vi "Event Handler.vi"(8 "error in (no error)":errorcluster, 10 "Stop Event Handler":refnum<user-event>, 11 "TreeDirectory in":refnum<class "TreeDirectory.lvclass">) -> (0 "error out":errorcluster)   [LabVIEW 2015, in "TreeDirectory.lvclass"]
doc: "The <b>Event Handler VI</b> is a dynamic dispatch VI that should be overwritten if events are needed to create the enhanced QControl. \n\nBy inheriting from the main Control.lvclass the overwritten <b>Event Handler VI</b> will be launched asynchronously in the initialization of the QControl.\n<b> </b> <b> </b>\n©2016 Q Software Innovations, LLC (QSI)\nwritten by Quentin Alldredge\nproduced in LabVIEW 2015\n\nsupport@qsoftwareinnovations.com\nwww.qsoftwareinnovations.com\n\nAll rights reserved.\n\nRedistribution and use in source and binary forms, with or without modification, are permitted provided that the following conditions are met:\n\n * Redistributions of source code must retain the above copyright notice, this list of conditions and the following disclaimer.\n * Redistributions in binary form must reproduce the above copyright notice, this list of conditions and the following disclaimer in the documentation and/or other materials provided with the distribution.\n * Neither the name of Q Software Innovations, LLC. nor the names of its contributors may be used to endorse or promote products derived from this software without specific prior written permission.\n\nTHIS SOFTWARE IS PROVIDED BY THE COPYRIGHT HOLDERS AND CONTRIBUTORS \"AS IS\" AND ANY EXPRESS OR IMPLIED WARRANTIES, INCLUDING, BUT NOT LIMITED TO, THE IMPLIED WARRANTIES OF MERCHANTABILITY AND FITNESS FOR A PARTICULAR PURPOSE ARE DISCLAIMED. IN NO EVENT SHALL THE COPYRIGHT OWNER OR CONTRIBUTORS BE LIABLE FOR ANY DIRECT, INDIRECT, INCIDENTAL, SPECIAL, EXEMPLARY, OR CONSEQUENTIAL DAMAGES (INCLUDING, BUT NOT LIMITED TO, PROCUREMENT OF SUBSTITUTE GOODS OR SERVICES; LOSS OF USE, DATA, OR PROFITS; OR BUSINESS INTERRUPTION) HOWEVER CAUSED AND ON ANY THEORY OF LIABILITY, WHETHER IN CONTRACT, STRICT LIABILITY, OR TORT (INCLUDING NEGLIGENCE OR OTHERWISE) ARISING IN ANY WAY OUT OF THE USE OF THIS SOFTWARE, EVEN IF ADVISED OF THE POSSIBILITY OF SUCH DAMAGE."
uses:
  TreeDirectory.lvclass
  TreeDirectory.lvclass/TreeDirectory.ctl
  TreeControl/TreeControl.lvclass
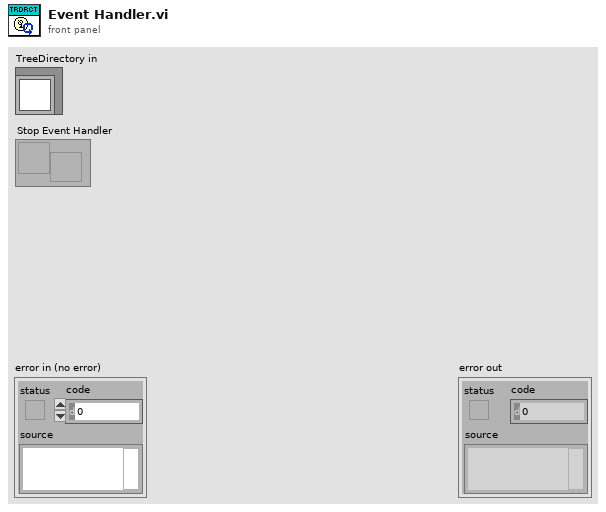
[diagram p1: front panel]
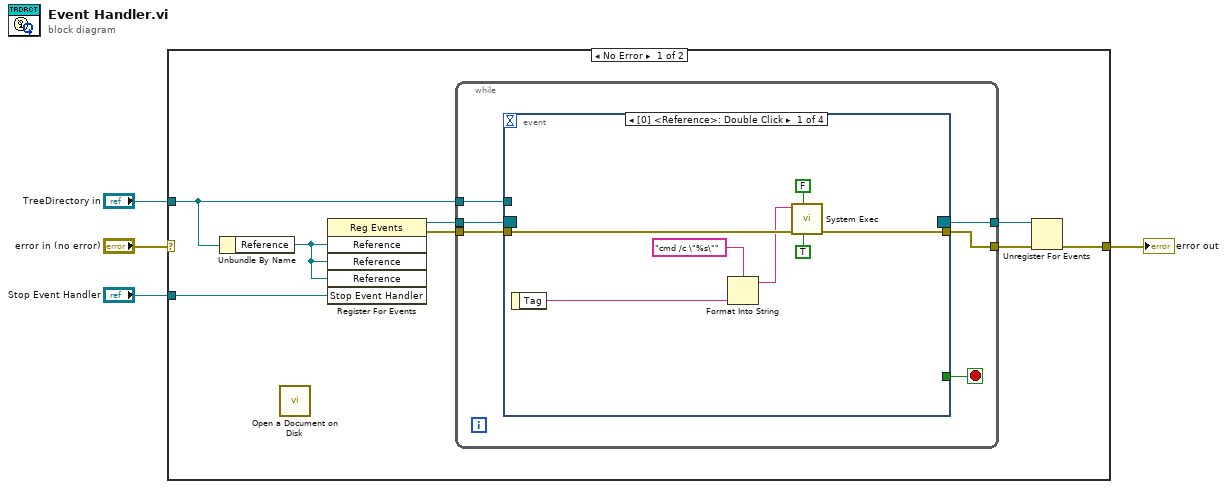
[diagram p0: block diagram]
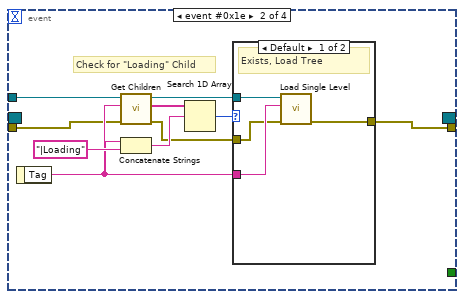
[diagram p2: hidden frame]
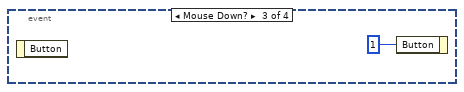
[diagram p4: hidden frame]
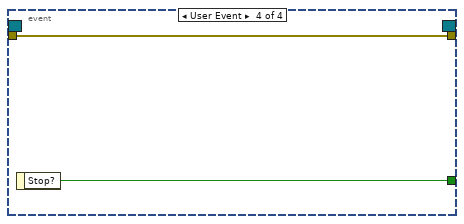
[diagram p5: hidden frame]
diagram:
  n1 = case shown="No Error" "error in (no error)" {
    selector: "error in (no error)" -> [_ w44]
    tunnel: [w9 w44] -> w3
    tunnel: "TreeDirectory in" -> [w7 _]
    tunnel: "Stop Event Handler" -> [w6 _]
    frame No Error {
      n2 = Unbundle By Name(w7) -> ("Reference"=w5:refnum<vi>)
      n3 = call <vilib>:"Open a Document on Disk.vi"() -> ()  [unwired: 7 in, 1 out]
      n4 = register-events(w5, w5, w5, w6) -> (reference out=w12:refnum<event-registration>, error out=w11:errorcluster)  [unwired: 2 in]
      n5 = while {
        tunnel: w12 -> [w18]
        tunnel: w11 -> [w16]
        tunnel: [w15] -> w10
        tunnel: [w13] -> w8
        tunnel: w7 -> [w17]
        stop <- w14 stop-if-true
        n6 = event shown="[0] <Reference>: Double Click" {
          selector: w18 -> [_ _ _ _]
          dyn-events: [_ _ _ _] -> w13
          timeout: _ -> [_ _ _ _]
          tunnel: w17 -> [_ w35 _ _]
          tunnel: w16 -> [w25 w28 _ w43]
          tunnel: [w24 w26 _ w43] -> w15
          tunnel: [_ _ _ w42] -> w14
          event Double Click {
            n7 = event-data() -> ("Tag"=w23:string)  [unwired: 1 in]
            n8 = Format Into String(format string="cmd /c \"%s\"", w23) -> (resulting string=w21:string)  [unwired: 2 in, 1 out]
            n9 = call <vilib>:"System Exec.vi"("run minimized? (F)"=TRUE, "wait until completion? (T)"=FALSE, "error in (no error)"=w25, "command line"=w21) -> ("error out"=w24:errorcluster)  [unwired: 4 in, 3 out]
          }
          event event #0x1e {
            # "Check for \"Loading\" Child"
            n10 = event-data() -> ("Tag"=w29:string)  [unwired: 1 in]
            n11 = call "Get Children.vi"("error in (no error)"=w28, "Tag"=w29, "Tree in"=w35) -> ("error out"=w27:errorcluster, "ChildrenTags[]"=w33:string[], "Tree out"=w30:refnum<class "TreeDirectory.lvclass">)  [unwired: 6 in]
            n12 = Concatenate Strings(w29, "|Loading" ("string")) -> (w32:string)
            n13 = Search 1D Array(1D array=w33, element=w32) -> (index of element=w31:i32)  [unwired: 1 in]
            n14 = case shown="Default" w31 {
              tunnel: w30 -> [w39 _]
              tunnel: w29 -> [w38 _]
              tunnel: w27 -> [w37 w40]
              tunnel: [w36 w40] -> w26
              frame Default {
                # "Exists, Load Tree"
                n15 = call "Load Single Level.vi"("error in (no error)"=w37, "Tag"=w38, "TreeDirectory in"=w39) -> ("error out"=w36:errorcluster)  [unwired: 7 in, 1 out]
              }
              frame -1 {
                # "DNE, Do Nothing"
              }
            }
          }
          event Mouse Down? {
            n16 = event-data() -> ()  [unwired: 1 in, 1 out]
            n17 = event-data("Button"=u16 1) -> ()  [unwired: 1 in, 1 out]
          }
          event User Event {
            n18 = event-data() -> ("Stop?"=w42:bool)  [unwired: 1 in]
          }
        }
      }
      n19 = Unregister For Events(event registration refnum=w8, error in=w10) -> (error out=w9:errorcluster)
    }
    frame Error {
    }
  }
  "error out" <- w3
